vi "ep_Get Waveform.vi"(6 "dt":dbl, 7 "t0":timestamp, 8 "error in (no error)":errorcluster, 9 "AI data":sgl[][](array[numeric]) format="%#.21g", 10 "physical channel indexes":u16[](array[numeric]), 11 "waveform in":waveform(sgl)[](array[waveform])) -> (0 "error out":errorcluster, 3 "waveform out":waveform(sgl)[](array[waveform]))   [LabVIEW 2014, in "NI_EP_Power Quality.lvlib"]
uses:
  <vilib>/addons/Electrical Power/PQ/NI_EP_Power Quality.lvlib
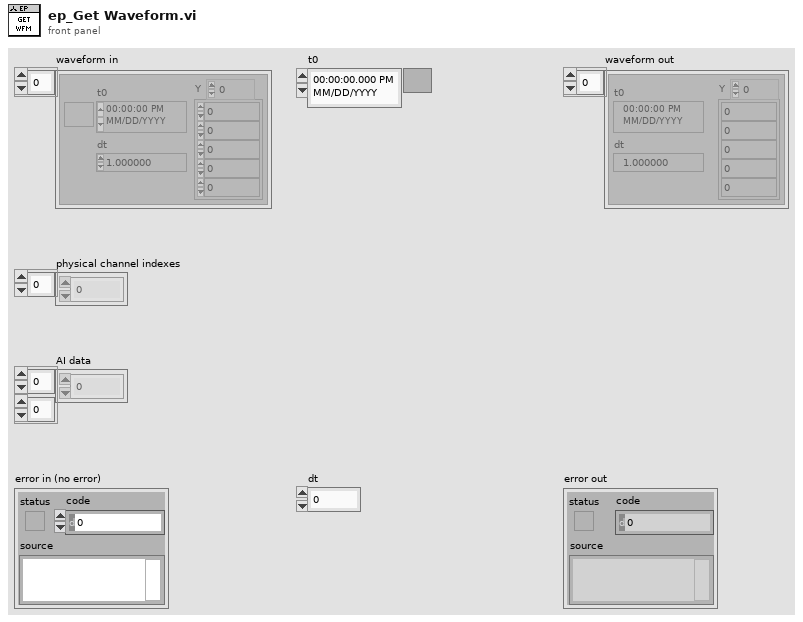
[diagram p1: front panel]
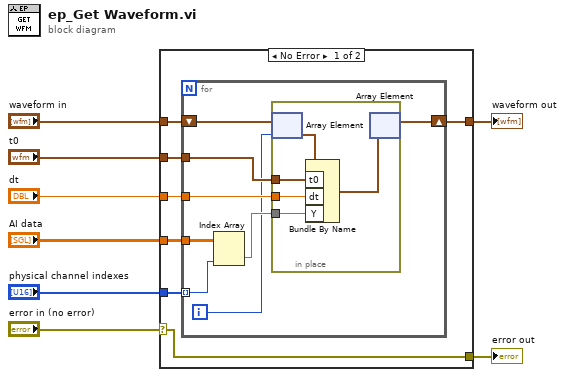
[diagram p0: block diagram]
diagram:
  n1 = case shown="No Error" "error in (no error)" {
    selector: "error in (no error)" -> [w9 w30]
    tunnel: "t0" -> [w15 _]
    tunnel: "dt" -> [w14 _]
    tunnel: "AI data" -> [w13 _]
    tunnel: [w12 w29] -> w5
    tunnel: "waveform in" -> [w11 w29]
    tunnel: "physical channel indexes" -> [w10 _]
    tunnel: [w9 w30] -> w1
    frame No Error {
      n2 = for {
        tunnel: w15 -> [w23]
        tunnel: w14 -> [w22]
        tunnel: w13 -> [w21]
        tunnel: w10 -> [w17] mode=indexing
        shift-right: [w16] -> w12
        shift-left: w11 -> [w19]
        i -> [w18]
        n3 = Index Array(array=w21, index (col)=w17) -> (element=w20:sgl[])  [unwired: 1 in]
        n4 = in-place {
          in-place-border: w20 -> [w25]
          in-place-border: w23 -> [w27]
          in-place-border: w22 -> [w26]
          n5 = in-place-array #1(w19, w18) -> (w28:waveform(sgl))
          n6 = Bundle By Name(cluster=w28, "t0"=w27, "dt"=w26, "Y"=w25) -> (w24:waveform(sgl))
          n7 = in-place-array #1(w24) -> (w16:waveform(sgl)[])  [unwired: 1 out]
        }
      }
    }
    frame Error {
    }
  }
  "waveform out" <- w5
  "error out" <- w1
